vi "diagStackMat.vi"(8 "error in (no error)":errorcluster, 9 "A1":dbl[][](array[numeric]), 10 "A0":dbl[][](array[numeric]), 11 "MatOper in":refnum<class "MatOper.lvclass">) -> (0 "error out":errorcluster, 2 "Diag Stack Matrix":dbl[][](array[numeric]), 3 "MatOper out":refnum<class "MatOper.lvclass">)   [LabVIEW 2016, in "OfcFunc.lvlib" / "MatOper.lvclass"]
doc: "Stack the matrixes (2D arrays actually) in the diagonal direction. For the inputs A1 and A2, the output matrix is:\n[A0, 0;\n 0, A1]."
uses:
  MatOper.lvclass
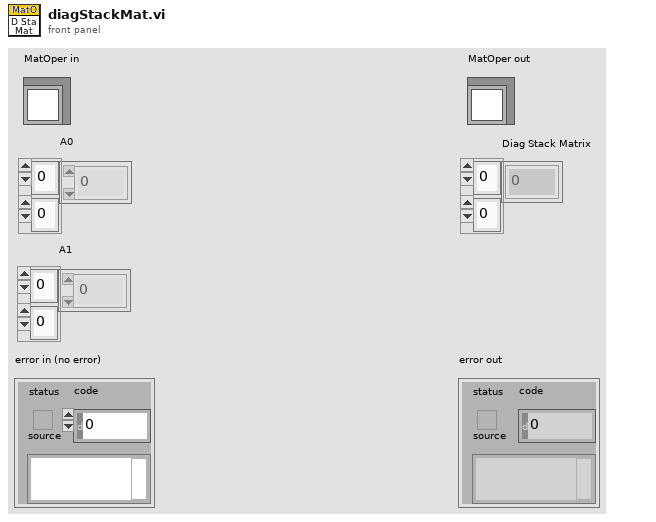
[diagram p1: front panel]
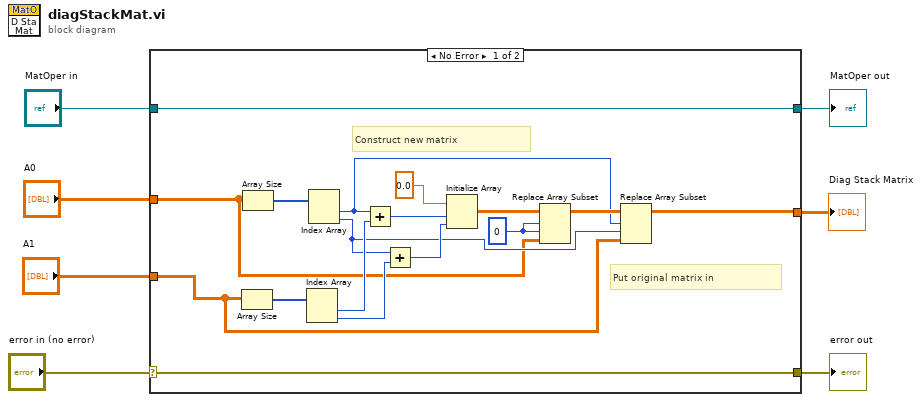
[diagram p0: block diagram]
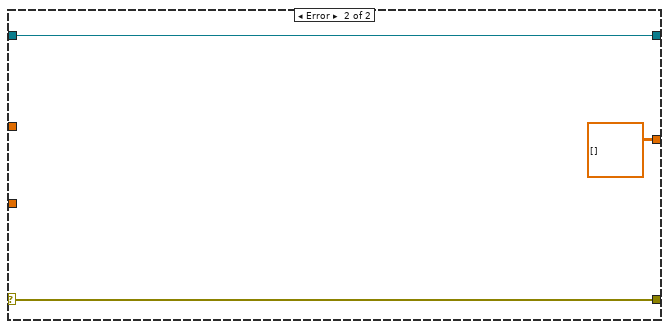
[diagram p2: hidden frame]
diagram:
  n1 = case shown="No Error" "error in (no error)" {
    selector: "error in (no error)" -> [w23 w27]
    tunnel: [w23 w27] -> w6
    tunnel: [w24 w26] -> w4
    tunnel: "MatOper in" -> [w24 w26]
    tunnel: "A0" -> [w10 _]
    tunnel: "A1" -> [w9 _]
    tunnel: [w8 dbl[][] []] -> w1
    frame No Error {
      w14 = 0 ("index (row)")
      # "Put original matrix in"
      # "Construct new matrix"
      n2 = Array Size(array=w9) -> (size(s)=w21:i32[])
      n3 = Array Size(array=w10) -> (size(s)=w22:i32[])
      n4 = Index Array(array=w21) -> (element #1=w20:i32, element #2=w19:i32)  [unwired: 2 in]
      n5 = Index Array(array=w22) -> (element #1=w12:i32, element #2=w11:i32)  [unwired: 2 in]
      n6 = Add(x=w12, y=w20) -> (x+y=w17:i32)
      n7 = Add(x=w11, y=w19) -> (x+y=w16:i32)
      n8 = Initialize Array(0.0 ("element"), w17, w16) -> (w15:dbl[][])
      n9 = Replace Array Subset(array=w15, new element=w10, index (row)=w14, index (col)=w14) -> (w13:dbl[][])
      n10 = Replace Array Subset(array=w13, new element=w9, index (row)=w12, index (col)=w11) -> (w8:dbl[][])
    }
    frame Error {
    }
  }
  "error out" <- w6
  "MatOper out" <- w4
  "Diag Stack Matrix" <- w1
